vi "映射处理.vi"() -> ()   [LabVIEW 2017]
uses:
  <vilib>/Utility/file.llb/Read Delimited Spreadsheet (string).vi
panel:
  out "Array":string[][](array[string])
  in  "file path (dialog if empty)":path
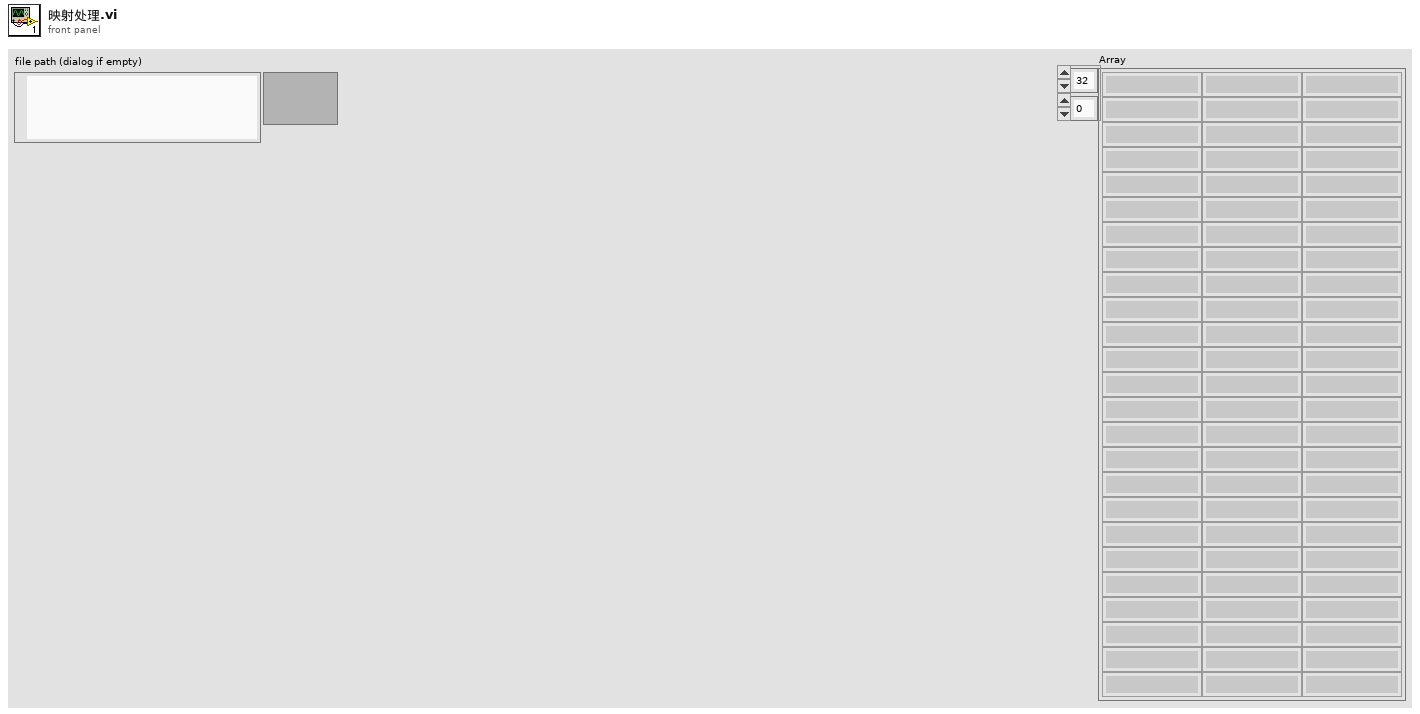
[diagram p1: front panel]
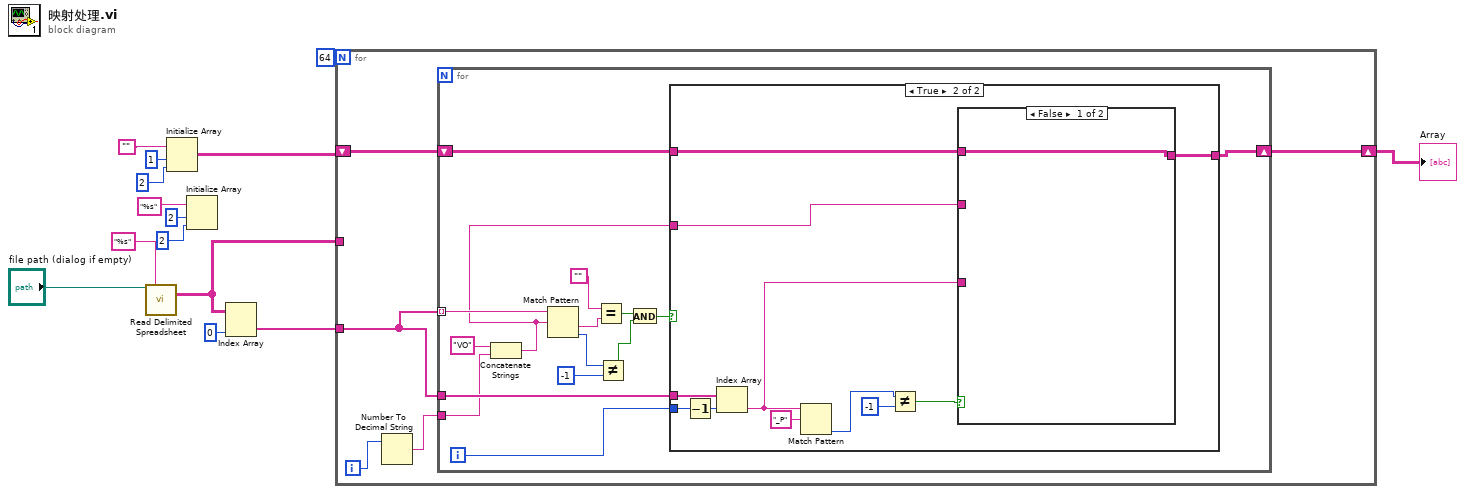
[diagram p0: block diagram]
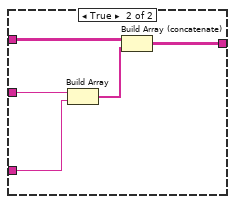
[diagram p3: hidden frame]
diagram:
  n1 = call-poly <vilib>:"Read Delimited Spreadsheet.vi"("file path (dialog if empty)"="file path (dialog if empty)", "format (%s)"="%s" ("format (%.3f)")) -> ("all rows"=w12:string[][])  [unwired: 8 in, 5 out]
  n2 = Initialize Array("", 1 ("dimension size"), 2 ("dimension size")) -> (w9:string[][])
  n3 = Initialize Array("%s" ("format (%.3f)"), 2 ("dimension size"), 2 ("dimension size")) -> ()  [unwired: 1 out]
  n4 = Index Array(array=w12, index (col)=0 ("disabled index (col)")) -> (element=w11:string[])  [unwired: 1 in]
  n5 = for {
    N: 64 -> [_]
    tunnel: w12 -> [_]
    tunnel: w11 -> [w19]
    shift-right: [w17] -> w2
    shift-left: w9 -> [w18]
    i -> [w16]
    n6 = Number To Decimal String(number=w16) -> (decimal integer string=w15:string)  [unwired: 1 in]
    n7 = for {
      tunnel: w19 -> [w34] mode=indexing
      tunnel: w19 -> [w31]
      shift-right: [w28] -> w17
      shift-left: w18 -> [w29]
      tunnel: w15 -> [w25]
      i -> [w30]
      n8 = Concatenate Strings("VO" ("search string"), w25) -> (w26:string)
      n9 = Match Pattern(string=w34, regular expression=w26) -> (after substring=w24:string, offset past match=w33:i32)  [unwired: 1 in, 2 out]
      n10 = Equal?(x="", y=w24) -> (x = y?=w22:bool)
      n11 = Not Equal?(x=w33, y=-1) -> (x != y?=w21:bool)
      n12 = And(x=w22, y=w21) -> (x .and. y?=w20:bool)
      n13 = case shown="True" w20 {
        tunnel: w31 -> [_ w46]
        tunnel: w30 -> [_ w45]
        tunnel: [w35 w39] -> w28
        tunnel: w29 -> [w35 w38]
        tunnel: w26 -> [_ w37]
        frame False {
        }
        frame True {
          n14 = Decrement(x=w45) -> (x-1=w44:i32)
          n15 = Index Array(array=w46, index=w44) -> (element=w36:string)
          n16 = Match Pattern(string=w36, regular expression="_P") -> (offset past match=w41:i32)  [unwired: 1 in, 3 out]
          n17 = Not Equal?(x=w41, y=-1) -> (x != y?=w40:bool)
          n18 = case shown="False" w40 {
            tunnel: [w47 w52] -> w39
            tunnel: w38 -> [w47 w51]
            tunnel: w37 -> [_ w50]
            tunnel: w36 -> [_ w49]
            frame False {
            }
            frame True {
              n19 = Build Array(w50, w49) -> (w48:string[])
              n20 = Build Array (concatenate)(w51, w48) -> (w52:string[][])
            }
          }
        }
      }
    }
  }
  "Array" <- w2
